vi "servo.vi"() -> ()   [LabVIEW 2020]
uses:
  <vilib>/High Genius/HG_WSI_Tookit/Dependencies/Library/PWM/PWM.lvclass
  C:/Program Files (x86)/National Instruments/LabVIEW 2020/vi.lib/High Genius/HG_WSI_Tookit/Dependencies/Library/HG_LIB/HG_LIB.lvclass
  <vilib>/Platform/TimedLoop/XDataNode/timing_clust.ctl
  <vilib>/Platform/TimedLoop/XDataNode/nitl_modes.ctl
  <vilib>/Platform/TimedLoop/XDataNode/wakeup.ctl
  <vilib>/platform/TimedLoop/XDataNode/XDataNode.xnode
  <vilib>/Platform/TimedLoop/XDataNode/XDNodeRunTimeDep.lvlib
  <vilib>/High Genius/HG_WSI_Tookit/Dependencies/Library/HG_LIB/HG_LIB.lvclass
panel:
  in  "Knob":dbl(knob) scale=0.0..2.0
  in  "stop":bool
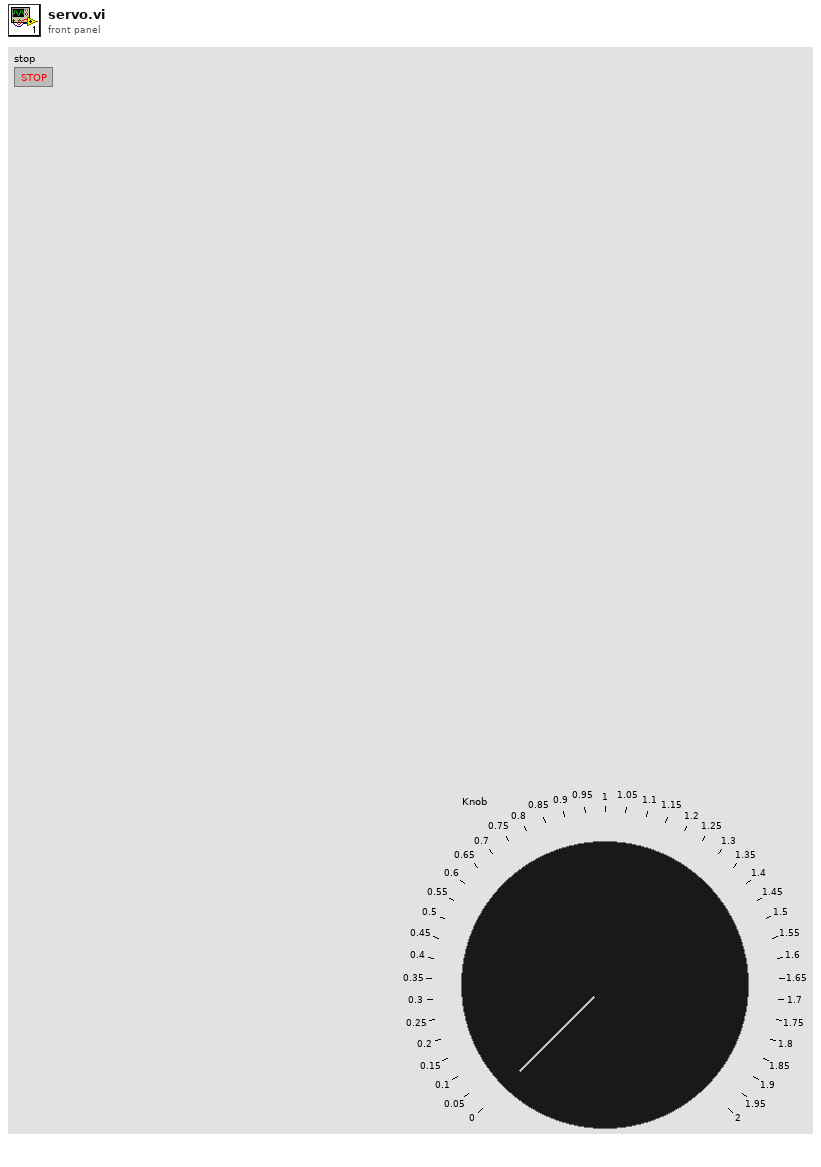
[diagram p1: front panel]
types:
  T1 = enum16{"DI", "DO", "AI", "Pulse", "PWM", "ISQ", "ENC", "CAN", "IIC", "IMU"}
  T2 = enum16{"0", "1", "2", "3", "4", "5", "6", "7", "8", "9", "10", "11", "12", "13", "14", "15", "16", "17", "18", "19", "20", "21", "22", "23", "24", "25"}
  T3 = typedef "XDNodeRunTimeDep.lvlib/timing_clust.ctl" = cluster{"Expected End [f-1]":u64, "Actual End [f-1]":u64, "Finished Late? [f-1]":bool, "Expected End [i-1]":u64, "Actual End [i-1]":u64, "Finished Late? [i-1]":bool, "Expected Start [i]":u64, "Actual Start [i]":u64, "Expected Start [f]":u64, "Actual Start [f]":u64, "Source Name":string, "Structure Name":string, "Period":i64, "Deadline":i64, "Offset":i64, "Start":i64, "Priority":i32, "Timeout":i32, "Mode":T4, "Wakeup Reason":T5, "Error":errorcluster, "Source Type":string, "Secondary Source Type":string, "Global End Time":u64, "Global Start Time":u64, "Frame Duration":u64, "Iteration Duration":u64, "Assigned CPU":i32, "I/O Scan Engine Mode":u32}
  T4 = typedef "XDNodeRunTimeDep.lvlib/nitl_modes.ctl" = enum32{"No Change", "Process missed periods, maintain original phase", "Discard missed periods, maintain original phase", "Process missed periods, ignore original phase", "Discard missed periods, ignore original phase"}
  T5 = typedef "XDNodeRunTimeDep.lvlib/wakeup.ctl" = enum32{"Normal", "Aborted", "Asynchronous wakeup", "Timing source error", "Timed loop error", "Timeout"}
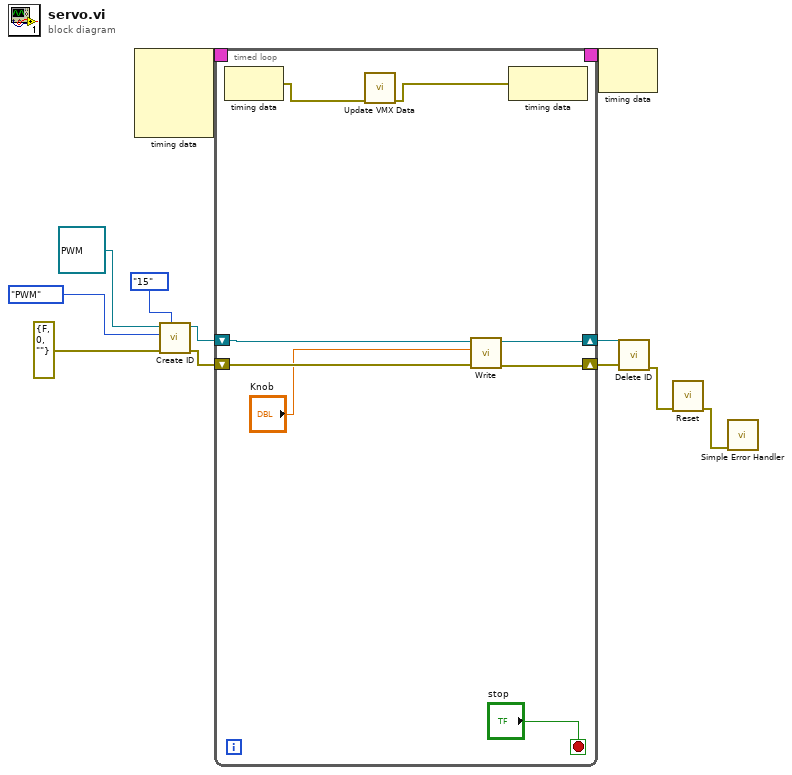
[diagram p0: block diagram]
diagram:
  n1 = node-c288() -> (w12:T3)  [unwired: 4 in]
  n2 = call <vilib>:"Create ID.vi"("NO"=T2."15", "error in (no error)"=errorcluster {"status"=FALSE, "code"=0, "source"=""}, "Function"=T1."PWM", "HG_LIB in"=refnum<class "PWM.lvclass"> refnum ("VMX Library.lvlib:PWM.lvclass")) -> ("error out"=w6:errorcluster, "HG_LIB out"=w7:refnum<class "PWM.lvclass">)  [unwired: 6 in]
  n3 = timed-loop {
    timing: w12 -> [_]
    timing-out: [_] -> w11
    shift-right: [w16] -> w1
    shift-left: w7 -> [w17]
    shift-right: [w15] -> w5
    shift-left: w6 -> [w14]
    stop <- "stop" stop-if-true
    n4 = node-c288() -> (w20:errorcluster)  [unwired: 1 in]
    n5 = call <vilib>:"Update VMX Data.vi"("error in (no error)"=w20) -> ("error out"=w19:errorcluster)  [unwired: 10 in]
    n6 = call <vilib>:"Write.vi"("error in (no error)"=w14, "PWM"="Knob", "PWM in"=w17) -> ("error out"=w15:errorcluster, "PWM out"=w16:refnum<class "PWM.lvclass">)  [unwired: 7 in]
    n7 = node-c288(w19) -> ()  [unwired: 1 out]
  }
  n8 = node-c288(w11) -> ()  [unwired: 1 out]
  n9 = call <vilib>:"Delete ID.vi"("error in (no error)"=w5, "HG_LIB in"=w1) -> ("error out"=w4:errorcluster)  [unwired: 8 in, 1 out]
  n10 = call <vilib>:"Reset.vi"("error in (no error)"=w4) -> ("error out"=w3:errorcluster)  [unwired: 10 in]
  n11 = call <vilib>:"Simple Error Handler.vi"("error in (no error)"=w3) -> ()  [unwired: 4 in, 5 out]
